vi "Process.vi"(8 "error in":errorcluster, 11 "Measurement.PhotocurrentMapping":refnum<class "Measurement.PhotocurrentMapping.lvclass">) -> (0 "error out":errorcluster, 3 "Measurement.PhotocurrentMapping out":refnum<class "Measurement.PhotocurrentMapping.lvclass">)   [LabVIEW 2017, in "Measurement.PhotocurrentMapping.lvclass"]
doc: "---------------------------------------------------------------\nJKI State Machine Objects™\nhttp://jki.net/state-machine-objects/\nCopyright (C) 2005-2015, JKI <info@jki.net>\nALL RIGHTS RESERVEDJKI State Machine Objects (SMO) 1.0.0.5\nJKI - JKI\nCopyright (c) 2016, JKI"
uses:
  Measurement.PhotocurrentMapping.lvclass
  D:/Program Files (x86)/National Instruments/LabVIEW 2017/vi.lib/JKI/JKI SMO/SMO/SMO.lvclass
  D:/upwork/Laser Measurement Tool/Laser/project/Subsystems/Measurement/Measurement.lvclass
  <vilib>/JKI/JKI SMO/SMO/Typedefs/Parent Call--Enum.ctl
  Measurement/Typedefs/Measurement.State--Enum.ctl
  Typedefs/Measurement.PhotocurrentMapping.State--Enum.ctl
  Typedefs/Results--Cluster.ctl
  Typedefs/Grid--Cluster.ctl
  Typedefs/Position--Cluster.ctl
  Typedefs/Measurement.PhotocurrentMapping.Measured--Data.ctl
  Measurement/Typedefs/PublicEvents--Measurement.Finished.ctl
  Measurement/Typedefs/PublicEvents--Measurement.Initialized.ctl
  Measurement/Typedefs/PublicEvents--Measurement.Escaped.ctl
  <vilib>/Analysis/baseanly.llb/Mean (DBL).vi
  SMU/SMU.lvclass
  D:/upwork/Laser Measurement Tool/Laser/project/Subsystems/MeasuringDevice/MeasuringDevice.lvclass
  LIA/LIA.lvclass
  Measurement/Measurement.lvclass
  <vilib>/JKI/JKI SMO/SMO/SMO.lvclass
  MeasuringDevice/MeasuringDevice.lvclass
  <vilib>/Analysis/NI_AALBase.lvlib
  XYStage/XYStage.lvclass
panel:
  # "Measurement.Photocurrent Mapping\nProcess.vi"
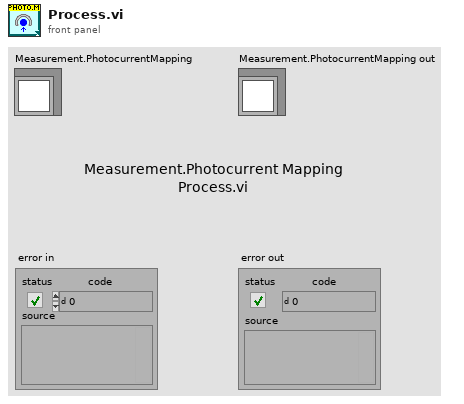
[diagram p1: front panel]
types:
  T1 = typedef "SMO.lvclass/Parent Call--Enum.ctl" = enum16{"Allows parent to run", "Does not request parent to run"}
  T2 = typedef "Measurement.lvclass/Measurement.State--Enum.ctl" = enum16{"Uninitialized", "Initialized", "Started", "Paused", "Stopped"}
  T3 = typedef "Measurement.PhotocurrentMapping.lvclass/Measurement.PhotocurrentMapping.State--Enum.ctl" = enum16{"Stoppped", "Wait for Postition set", "Wait for Measurements"}
  T4 = enum32{"invalid app kind", "Development System", "Run Time System", "Student Edition", "Embedded LabVIEW", "Evaluation", "Custom"}
  T5 = typedef "Measurement.PhotocurrentMapping.lvclass/Position--Cluster.ctl" = cluster{"X":dbl, "Y":dbl}
  T6 = enum32{"Invalid", "Standard", "Closed", "Hidden", "Minimized", "Maximized"}
  T7 = typedef "Measurement.lvclass/PublicEvents--Measurement.Finished.ctl" = bool
  T8 = typedef "Measurement.lvclass/PublicEvents--Measurement.Initialized.ctl" = bool
  T9 = typedef "Measurement.PhotocurrentMapping.lvclass/Dependencies--Cluster.ctl" = cluster{"SMU":refnum<class "SMU.lvclass">, "LIA":refnum<class "LIA.lvclass">, "XYStage":refnum<class "XYStage.lvclass">}
  T10 = typedef "Measurement.PhotocurrentMapping.lvclass/Configuration--Cluster.ctl" = cluster{"Measurement.Type":T11, "Hardware":T12, "Measurement":T19}
  T11 = typedef "Measurement.lvclass/Measurement.Type--Enum.ctl" = enum16{"Free", "I/V Curve", "Wavelength sweeping", "Photocurrent mapping"}
  T12 = typedef "Measurement.PhotocurrentMapping.lvclass/Configuration.Hardware--Cluster.ctl" = cluster{"SMU":T13, "LIA":T15, "XYStage":T17}
  T13 = typedef "Measurement.lvclass/Configuration.SMU--Cluster.ctl" = cluster{"Enable":bool, "SMU Model":string, "Configuration":T14}
  T14 = typedef "SMU.lvclass/Configuration--Cluster.ctl" = cluster{"VISA Resource":string, "Channel":string}
  T15 = typedef "Measurement.lvclass/Configuration.LIA--Cluster.ctl" = cluster{"Enable":bool, "LIA Model":string, "Configuration":T16}
  T16 = typedef "LIA.lvclass/Configuration--Cluster.ctl" = cluster{"VISA Resource":string}
  T17 = typedef "Measurement.lvclass/Configuration.XYStage--Cluster.ctl" = cluster{"Enable":bool, "XYStage Model":string, "Configuration":T18}
  T18 = typedef "XYStage.lvclass/Configuration--Cluster.ctl" = cluster{"Serial Number":string, "X Axis":string, "Y Axis":string, "Real-World Units":string, "Counts per Unit":u32}
  T19 = typedef "Measurement.PhotocurrentMapping.lvclass/Configuration.Measurement--Cluster.ctl" = cluster{"X":T20, "Y":T20, "Accumulation":u16}
  T20 = typedef "Measurement.PhotocurrentMapping.lvclass/Configuration.Axis--Cluster.ctl" = cluster{"Start, units":dbl, "Stop, units":dbl, "Step, units":dbl}
  T21 = typedef "Measurement.PhotocurrentMapping.lvclass/Results--Cluster.ctl" = cluster{"SMU Completed":bool, "LIA Completed":bool, "SMU Measurement":dbl, "LIA Measurement":dbl, "XYStage Completed":bool}
  T22 = typedef "Measurement.PhotocurrentMapping.lvclass/Grid--Cluster.ctl" = cluster{"Positions":T5[][], "X Index":i32, "Y Index":i32, "X Count":u32, "Y Count":u32}
  T23 = cluster{"Core":cluster{"Current VI Reference":refnum<vi>, "Close Panel on Exit?":bool, "error":errorcluster}, "Self Reference":refnum<class "Measurement.PhotocurrentMapping.lvclass">, "Dependencies":T9, "Configuration":T10, "Initialized":bool, "Meas State":T2, "P-Map State":T3, "Next Step":string, "Results":T21, "Grid":T22}
  T24 = cluster{"Current VI Reference":refnum<vi>, "Close Panel on Exit?":bool, "error":errorcluster}
  T25 = typedef "Measurement.PhotocurrentMapping.lvclass/Measurement.PhotocurrentMapping.Measured--Data.ctl" = cluster{"Current, A":dbl, "Magnitude":dbl}
  T26 = typedef "SMO.lvclass/Protected Events.ctl" = cluster{"StopProcesses":refnum<user-event>, "AbortProcesses":refnum<user-event>, "Config Changed":refnum<user-event>, "Dependency":refnum<user-event>}
  T27 = cluster{"Event Registration Refnum":refnum<event-registration>, "Measurement Protected Events":refnum<event-registration>, "SMU Public Events":refnum<event-registration>, "LIA Public Events":refnum<event-registration>, "XYStage Public Events":refnum<event-registration>}
  T28 = typedef "Measurement.lvclass/PublicEvents--Measurement.Escaped.ctl" = bool
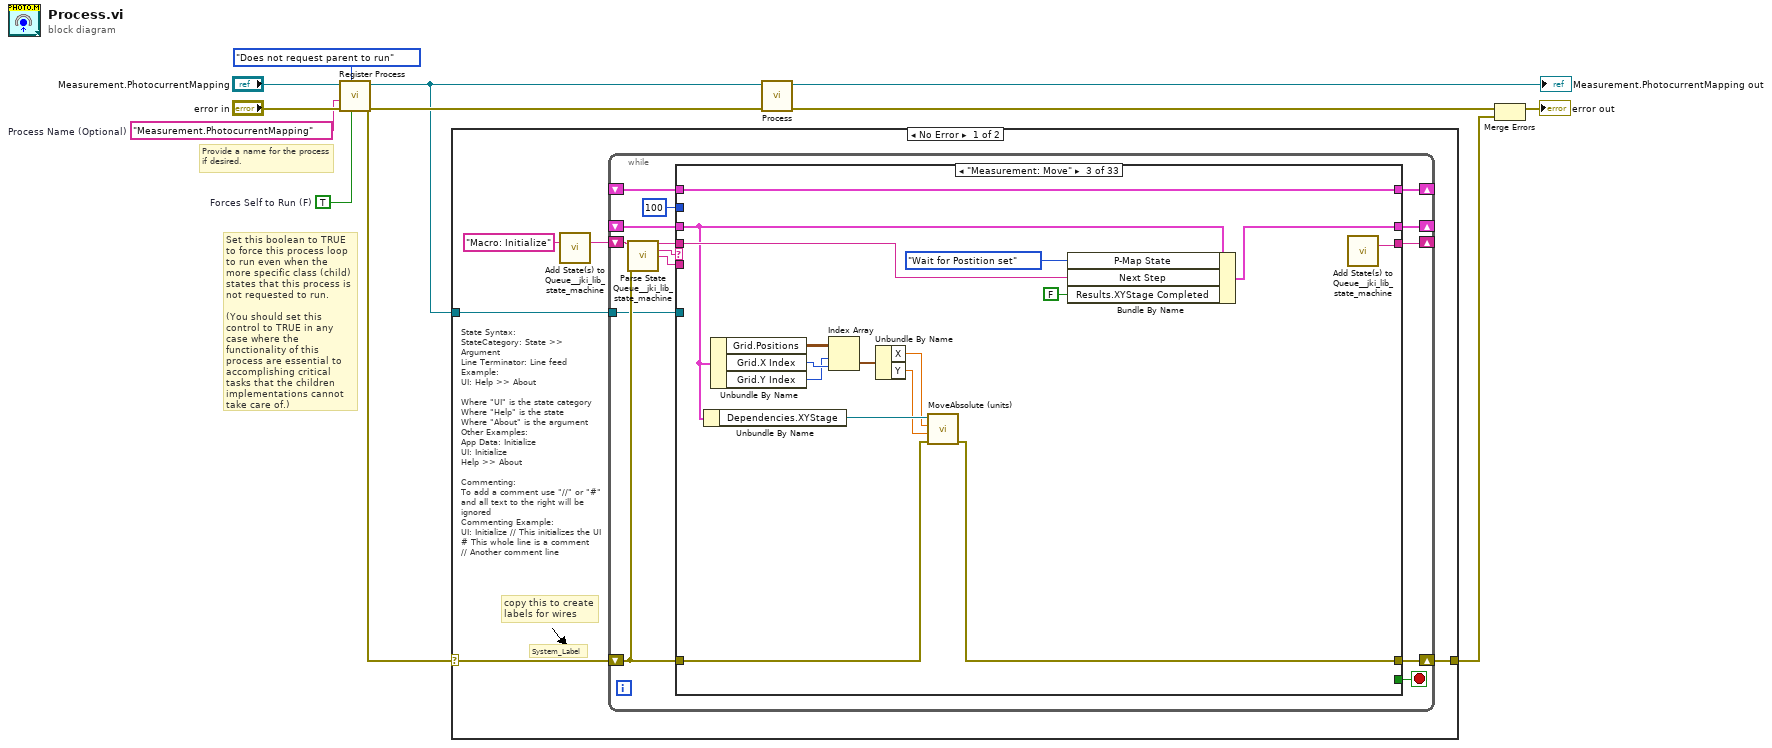
[diagram p0: block diagram]
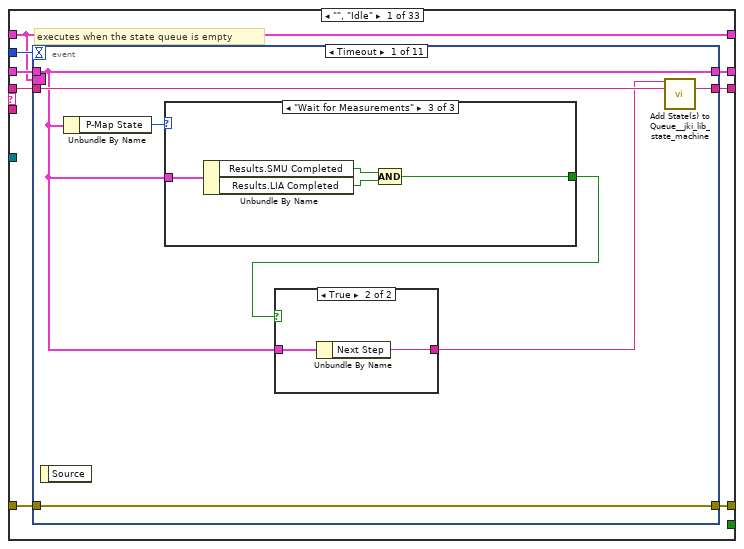
[diagram p2: hidden frame]
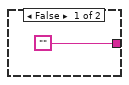
[diagram p3: hidden frame]
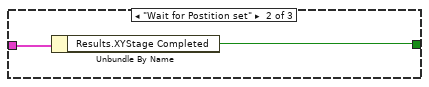
[diagram p5: hidden frame]
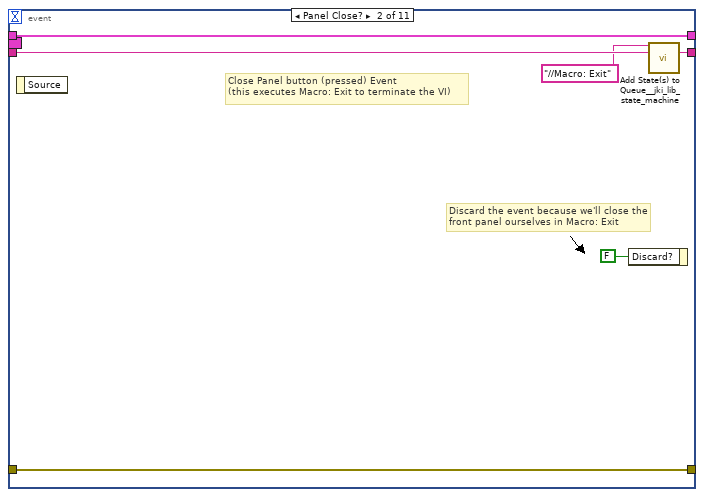
[diagram p6: hidden frame]
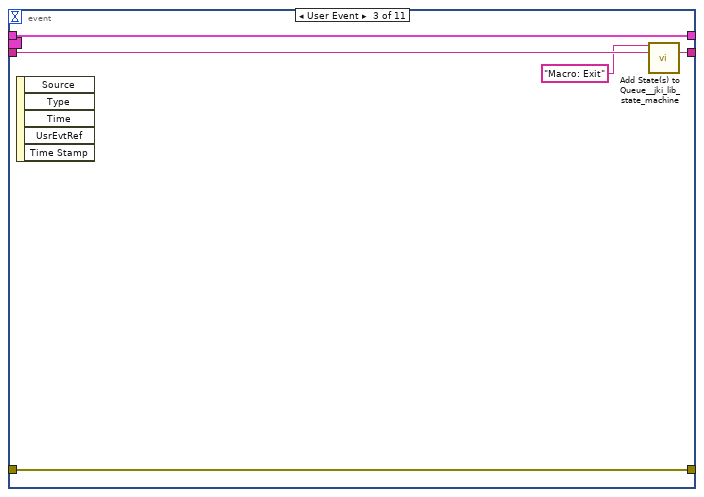
[diagram p7: hidden frame]
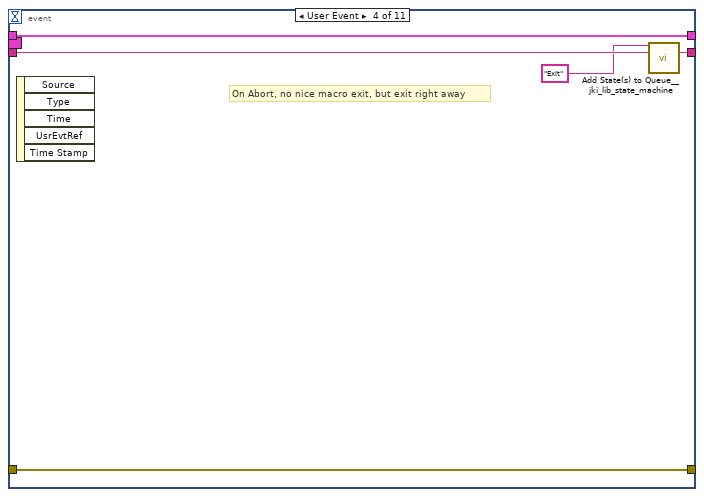
[diagram p8: hidden frame]
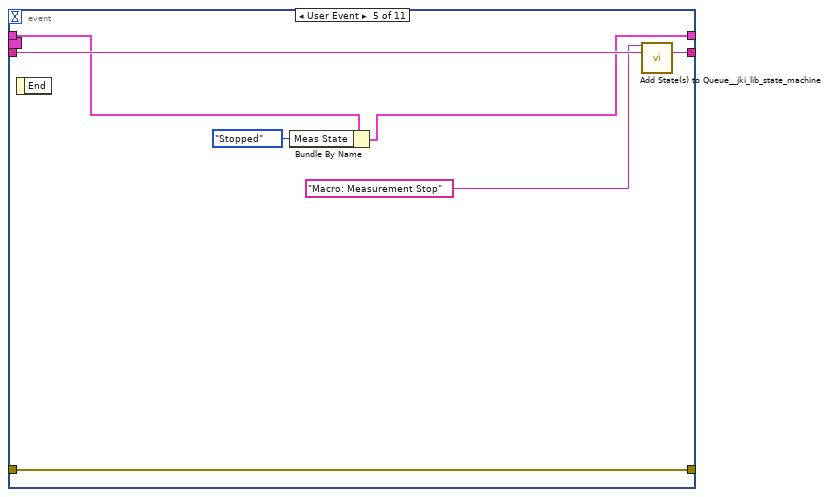
[diagram p9: hidden frame]
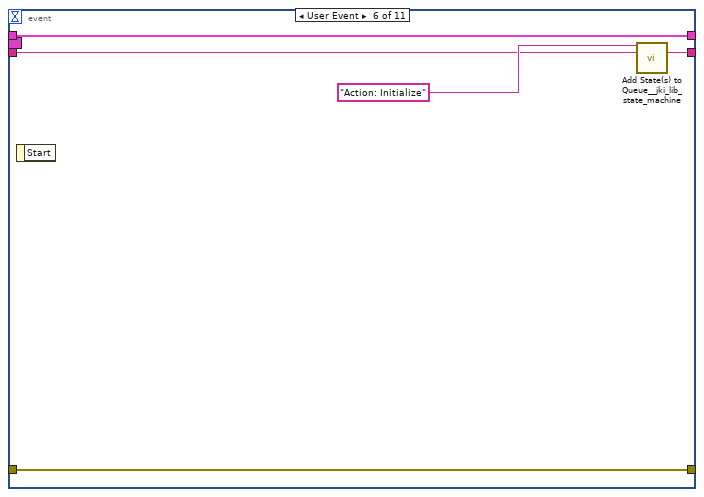
[diagram p10: hidden frame]
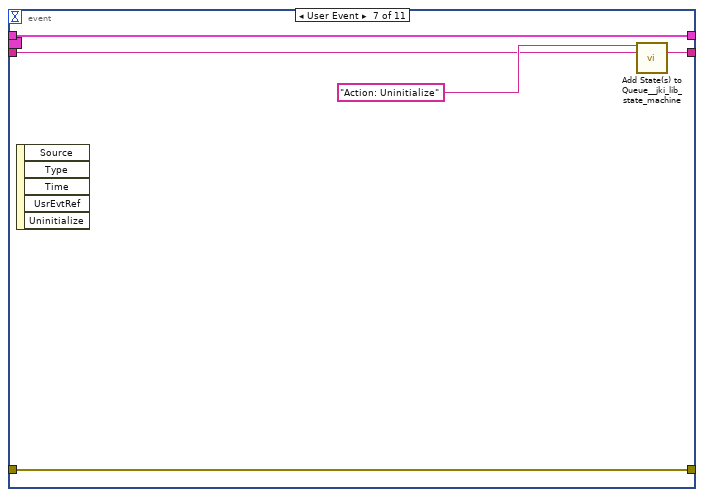
[diagram p11: hidden frame]
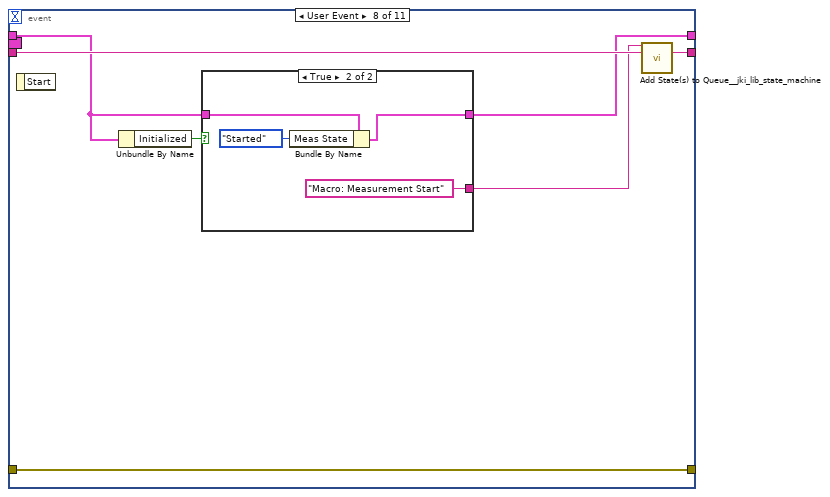
[diagram p12: hidden frame]
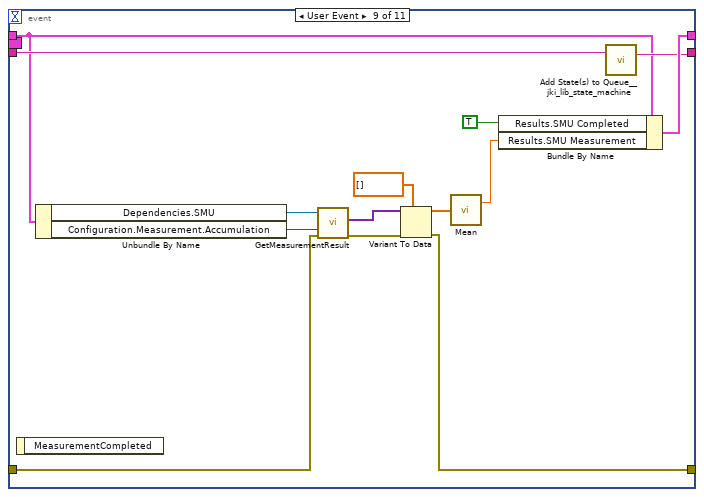
[diagram p14: hidden frame]
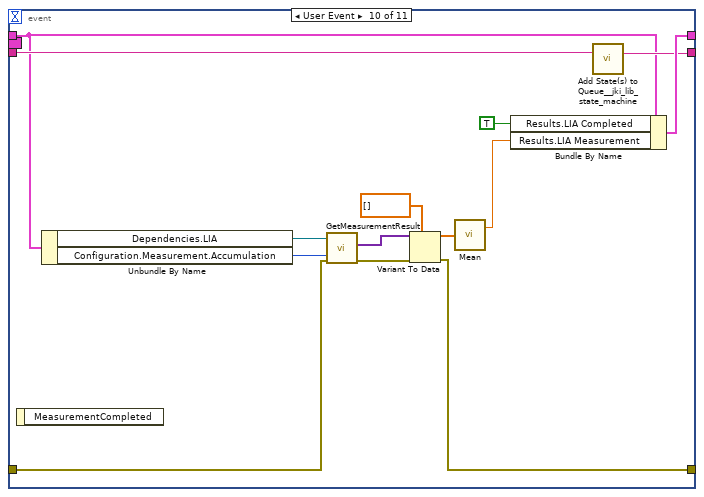
[diagram p15: hidden frame]
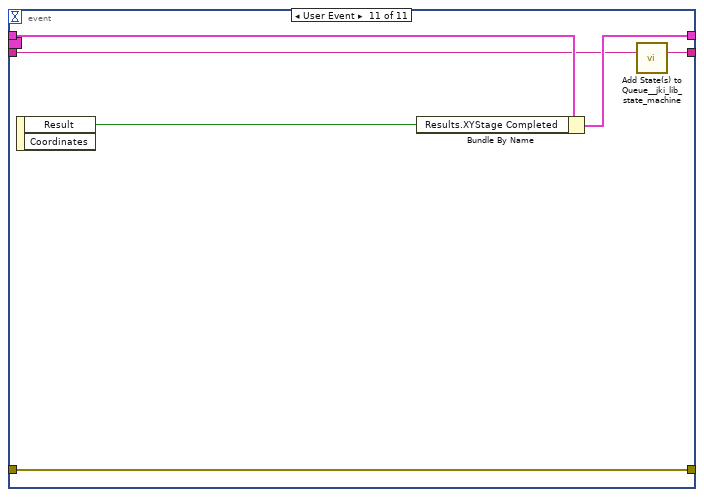
[diagram p16: hidden frame]
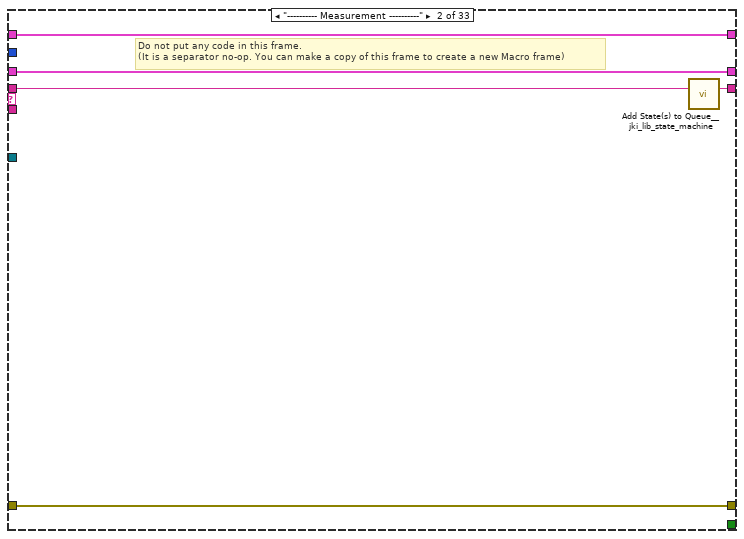
[diagram p17: hidden frame]
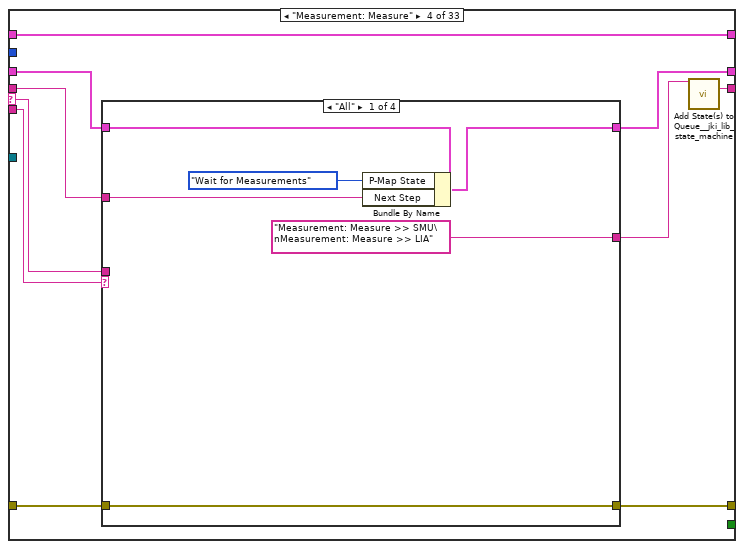
[diagram p18: hidden frame]
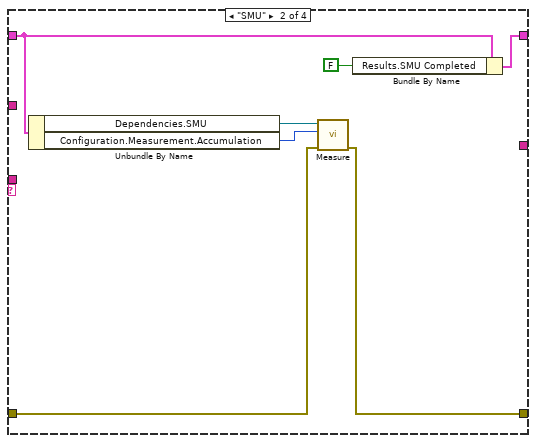
[diagram p19: hidden frame]
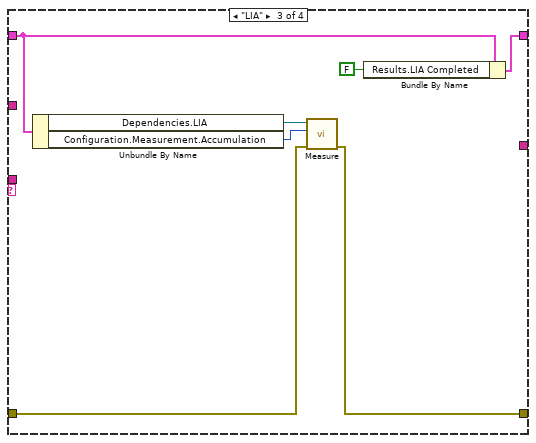
[diagram p20: hidden frame]
diagram:
  w2 = TRUE  # Forces Self to Run (F)
  w1 = "Measurement.PhotocurrentMapping"  # Process Name (Optional)
  # "Provide a name for the process\nif desired."
  # "Set this boolean to TRUE to force this process loop to run even when the more specific class (child) states that this process is not requested to run.\n\n(You should set this control to TRUE in any case where the functionality of this process are essential to accomplishing critical tasks that the children implementations cannot take care of.)"
  n1 = call <vilib>:"Register Process.vi"("Forces Self to Run (F)"=w2, "Parent Call"=Parent_Call--Enum."Does not request parent to run", "error in (no error)"="error in", "Process Name (optional)"=w1, "SMO"="Measurement.PhotocurrentMapping") -> ("error out"=w8:errorcluster, "SMO out"=w7:refnum<class "Measurement.PhotocurrentMapping.lvclass">)  [unwired: 5 in]
  n2 = case shown="No Error" w8 {
    selector: w8 -> [w13 w561]
    tunnel: w7 -> [w14 _]
    tunnel: [w12 w561] -> w4
    frame No Error {
      # "State Syntax:\nStateCategory: State >> Argument\nLine Terminator: Line feed\nExample:\nUI: Help >> About\n\nWhere \"UI\" is the state category\nWhere \"Help\" is the state\nWhere \"About\" is the argument\nOther Examples:\nApp Data: Initialize\nUI: Initialize\nHelp >> About\n\nCommenting:\nTo add a comment use \"//\" or \"#\" and all text to the right will be ignored\nCommenting Example:\nUI: Initialize // This initializes the UI\n# This whole line is a comment\n// Another comment line"
      # "copy this to create labels for wires"
      # "System_Label"
      n3 = call <vilib>:"Add State(s) to Queue__jki_lib_state_machine.vi"("State(s) in (\"\")"="Macro: Initialize") -> ("States Out"=w16:string)  [unwired: 14 in]
      n4 = while {
        shift-right: [w23] -> _
        shift-left: _ -> [w22]
        shift-right: [w26] -> w12
        shift-left: w13 -> [w20]
        shift-right: [w25] -> _
        shift-left: w16 -> [w27]
        tunnel: w14 -> [w19]
        shift-right: [w18] -> _
        shift-left: _ -> [w17]
        stop <- w24 stop-if-true
        n5 = call <vilib>:"Parse State Queue__jki_lib_state_machine.vi"("State Queue"=w27, "Error In (no error)"=w20) -> ("Remaining States"=w29:string, "Current State"=w30:string, "Arguments"=w28:string)  [unwired: 11 in]
        n6 = case shown="\"Measurement: Move\"" w30 {
          selector: w30 -> [_ _ _ w156 _ _ w232 _ _ _ _ _ _ _ _ _ _ _ _ _ _ _ _ _ _ _ _ _ _ _ _ _ _]
          tunnel: w29 -> [w38 w138 w151 w155 w209 w230 w236 w255 w270 w276 w281 w302 w309 w329 w346 w351 w358 w374 w413 w418 w427 w441 w447 w460 w465 w476 w481 w503 w509 w514 w527 w545 w560]
          tunnel: w28 -> [_ _ _ w162 _ _ _ _ _ _ _ _ _ _ _ _ w352 w368 _ _ _ _ _ _ _ _ _ _ _ _ _ _ _]
          tunnel: w22 -> [w36 w135 w150 w158 w198 w227 w234 w246 w261 w272 w278 _ w304 w316 w343 w349 w356 w370 w410 w415 w423 w432 w443 w452 w462 w473 w478 w485 w507 w512 w519 w536 w557]
          tunnel: [w35 w136 w141 w159 w207 w228 w238 w252 w263 w271 w279 w290 w305 w327 w344 w348 w353 w371 w404 w416 w425 w439 w445 w449 w463 w467 w479 w498 w505 w510 w516 w540 w554] -> w26
          tunnel: w20 -> [w34 w136 w142 w160 w207 w228 w237 w252 w258 _ w279 w299 w306 w327 w344 w348 w354 w372 w405 w416 w425 w439 w445 w450 w463 w468 w479 w486 w505 w510 w523 w541 w555]
          tunnel: [w37 w137 w139 w164 w208 w229 w235 w254 w269 w275 w280 w301 w308 w328 w345 w350 w357 w373 w412 w417 w426 w440 w446 w459 w464 w475 w480 w502 w508 w513 w526 w544 w559] -> w25
          tunnel: [_ _ _ _ _ _ _ _ _ TRUE _ _ _ _ _ _ _ _ _ _ _ _ _ _ _ _ _ _ _ _ _ _ _] -> w24
          tunnel: [w33 w135 w153 w157 w195 w227 w234 w253 w260 w272 w278 w300 w304 w315 w343 w349 w356 w370 w410 w415 w423 w432 w443 w453 w462 w473 w478 w485 w507 w512 w518 w539 w557] -> w23
          tunnel: 100 ("Timeout") -> [w32 _ _ _ _ _ _ _ _ _ _ _ _ _ _ _ _ _ _ _ _ _ _ _ _ _ _ _ _ _ _ _ _]
          tunnel: w19 -> [_ _ _ _ _ _ _ _ _ _ _ w297 _ _ _ _ _ _ _ _ _ _ _ _ _ _ _ _ _ _ w524 w542 w556]
          tunnel: [w31 w134 w154 w163 w206 w226 w231 w243 w268 w273 w277 w296 w303 w326 w342 w347 w355 w367 w411 w414 w424 w433 w444 w458 w461 w474 w477 w497 w506 w511 w525 w543 w558] -> w18
          tunnel: w17 -> [w31 w134 w154 w163 w206 w226 w231 w243 w268 w273 w277 w296 w303 w326 w342 w347 w355 w367 w411 w414 w424 w433 w444 w458 w461 w474 w477 _ w506 w511 w525 w543 w558]
          frame "", "Idle" {
            # "executes when the state queue is empty"
            n7 = event shown="[0] Timeout" {
              selector: w31 -> [_ _ _ _ _ _ _ _ _ _ _]
              dyn-events: _ -> [_ _ _ _ _ _ _ _ _ _ _]
              timeout: w32 -> [_ _ _ _ _ _ _ _ _ _ _]
              tunnel: w38 -> [w45 w60 w65 w70 w76 w78 w83 w93 w111 w125 w130]
              tunnel: [w44 w59 w64 w69 w77 w80 w85 w94 w112 w126 w131] -> w37
              tunnel: w36 -> [w40 w57 w62 w67 w73 w81 w86 w89 w110 w121 w133]
              tunnel: [w43 w58 w63 w68 w75 w82 w87 w92 w105 w119 w128] -> w35
              tunnel: w34 -> [w43 w58 w63 w68 w75 w82 w87 w92 w108 w120 w128]
              tunnel: [w40 w57 w62 w67 w72 w81 w86 w88 w113 w127 w132] -> w33
              event Timeout {
                n8 = event-data() -> ()  [unwired: 1 in, 1 out]
                n9 = Unbundle By Name(w40) -> ("P-Map State"=w42:T3)
                n10 = case shown="\"Wait for Measurements\"" w42 {
                  tunnel: w40 -> [_ w50 w54]
                  tunnel: [_ w49 w52] -> w41
                  frame "Stoppped", Default {
                  }
                  frame "Wait for Postition set" {
                    n11 = Unbundle By Name(w50) -> ("Results.XYStage Completed"=w49:bool)
                  }
                  frame "Wait for Measurements" {
                    n12 = Unbundle By Name(w54) -> ("Results.SMU Completed"=w53:bool, "Results.LIA Completed"=w51:bool)
                    n13 = Compound Arithmetic op=AND(w53, w51) -> (w52:bool)
                  }
                }
                n14 = case shown="True" w41 {
                  tunnel: w40 -> [_ w48]
                  tunnel: ["" w47] -> w39
                  frame False {
                  }
                  frame True {
                    n15 = Unbundle By Name(w48) -> ("Next Step"=w47:string)
                  }
                }
                n16 = call <vilib>:"Add State(s) to Queue__jki_lib_state_machine.vi"("State(s) in Front (\"\")"=w39, "State(s) in (\"\")"=w45) -> ("States Out"=w44:string)  [unwired: 13 in]
              }
              event Panel Close? {
                # "Discard the event because we'll close the front panel ourselves in Macro: Exit"
                # "Close Panel button (pressed) Event\n(this executes Macro: Exit to terminate the VI)"
                n17 = event-data() -> ()  [unwired: 1 in, 1 out]
                n18 = event-data("Discard?"=FALSE) -> ()  [unwired: 1 in, 1 out]
                n19 = call <vilib>:"Add State(s) to Queue__jki_lib_state_machine.vi"("State(s) in Front (\"\")"="//Macro: Exit", "State(s) in (\"\")"=w60) -> ("States Out"=w59:string)  [unwired: 13 in]
              }
              event User Event {
                n20 = event-data() -> ()  [unwired: 1 in, 5 out]
                n21 = call <vilib>:"Add State(s) to Queue__jki_lib_state_machine.vi"("State(s) in Front (\"\")"="Macro: Exit", "State(s) in (\"\")"=w65) -> ("States Out"=w64:string)  [unwired: 13 in]
              }
              event User Event {
                # "On Abort, no nice macro exit, but exit right away"
                n22 = event-data() -> ()  [unwired: 1 in, 5 out]
                n23 = call <vilib>:"Add State(s) to Queue__jki_lib_state_machine.vi"("State(s) in Front (\"\")"="Exit", "State(s) in (\"\")"=w70) -> ("States Out"=w69:string)  [unwired: 13 in]
              }
              event User Event {
                n24 = event-data() -> ()  [unwired: 1 in, 1 out]
                n25 = Bundle By Name(cluster=w73, "Meas State"=Measurement.State--Enum."Stopped") -> (w72:T23)
                n26 = call <vilib>:"Add State(s) to Queue__jki_lib_state_machine.vi"("State(s) in Front (\"\")"="Macro: Measurement Stop", "State(s) in (\"\")"=w76) -> ("States Out"=w77:string)  [unwired: 13 in]
              }
              event User Event {
                n27 = event-data() -> ()  [unwired: 1 in, 1 out]
                n28 = call <vilib>:"Add State(s) to Queue__jki_lib_state_machine.vi"("State(s) in Front (\"\")"="Action: Initialize", "State(s) in (\"\")"=w78) -> ("States Out"=w80:string)  [unwired: 13 in]
              }
              event User Event {
                n29 = event-data() -> ()  [unwired: 1 in, 5 out]
                n30 = call <vilib>:"Add State(s) to Queue__jki_lib_state_machine.vi"("State(s) in Front (\"\")"="Action: Uninitialize", "State(s) in (\"\")"=w83) -> ("States Out"=w85:string)  [unwired: 13 in]
              }
              event User Event {
                n31 = event-data() -> ()  [unwired: 1 in, 1 out]
                n32 = Unbundle By Name(w89) -> ("Initialized"=w90:bool)
                n33 = case shown="True" w90 {
                  tunnel: [_ "Macro: Measurement Start"] -> w91
                  tunnel: w89 -> [w95 w98]
                  tunnel: [w95 w96] -> w88
                  frame False {
                  }
                  frame True {
                    n34 = Bundle By Name(cluster=w98, "Meas State"=Measurement.State--Enum."Started") -> (w96:T23)
                  }
                }
                n35 = call <vilib>:"Add State(s) to Queue__jki_lib_state_machine.vi"("State(s) in Front (\"\")"=w91, "State(s) in (\"\")"=w93) -> ("States Out"=w94:string)  [unwired: 13 in]
              }
              event User Event {
                n36 = event-data() -> ()  [unwired: 1 in, 1 out]
                n37 = Unbundle By Name(w110) -> ("Dependencies.SMU"=w109:refnum<class "SMU.lvclass">, "Configuration.Measurement.Accumulation"=w101:u16)
                n38 = call "GetMeasurementResult.vi"("error in (no error)"=w108, "Count (1)"=w101, "MeasuringDevice in"=w109) -> ("error out"=w106:errorcluster, "Result"=w107:variant[])  [unwired: 6 in, 1 out]
                n39 = Variant To Data(error in=w106, type=dbl[] [], Variant=w107) -> (data=w103:dbl[], error out=w105:errorcluster)
                n40 = call-poly <vilib>:"Mean.vi"("X"=w103) -> ("mean"=w102:dbl)  [unwired: 1 out]
                n41 = Bundle By Name(cluster=w110, "Results.SMU Completed"=TRUE ("OPA Wavelength"), "Results.SMU Measurement"=w102) -> (w113:T23)
                n42 = call <vilib>:"Add State(s) to Queue__jki_lib_state_machine.vi"("State(s) in (\"\")"=w111) -> ("States Out"=w112:string)  [unwired: 14 in]
              }
              event User Event {
                n43 = event-data() -> ()  [unwired: 1 in, 1 out]
                n44 = Unbundle By Name(w121) -> ("Dependencies.LIA"=w124:refnum<class "LIA.lvclass">, "Configuration.Measurement.Accumulation"=w115:u16)
                n45 = call "GetMeasurementResult.vi"("error in (no error)"=w120, "Count (1)"=w115, "MeasuringDevice in"=w124) -> ("error out"=w122:errorcluster, "Result"=w123:variant[])  [unwired: 6 in, 1 out]
                n46 = Variant To Data(error in=w122, type=dbl[] [], Variant=w123) -> (data=w118:dbl[], error out=w119:errorcluster)
                n47 = call-poly <vilib>:"Mean.vi"("X"=w118) -> ("mean"=w116:dbl)  [unwired: 1 out]
                n48 = Bundle By Name(cluster=w121, "Results.LIA Completed"=TRUE ("OPA Wavelength"), "Results.LIA Measurement"=w116) -> (w127:T23)
                n49 = call <vilib>:"Add State(s) to Queue__jki_lib_state_machine.vi"("State(s) in (\"\")"=w125) -> ("States Out"=w126:string)  [unwired: 14 in]
              }
              event User Event {
                n50 = event-data() -> ("Result"=w129:bool)  [unwired: 1 in, 1 out]
                n51 = Bundle By Name(cluster=w133, "Results.XYStage Completed"=w129) -> (w132:T23)
                n52 = call <vilib>:"Add State(s) to Queue__jki_lib_state_machine.vi"("State(s) in (\"\")"=w130) -> ("States Out"=w131:string)  [unwired: 14 in]
              }
            }
          }
          frame "---------- Measurement ----------" {
            # "Do not put any code in this frame.\n(It is a separator no-op. You can make a copy of this frame to create a new Macro frame)"
            n53 = call <vilib>:"Add State(s) to Queue__jki_lib_state_machine.vi"("State(s) in (\"\")"=w138) -> ("States Out"=w137:string)  [unwired: 14 in]
          }
          frame "Measurement: Move" {
            n54 = Unbundle By Name(w150) -> ("Dependencies.XYStage"=w149:refnum<class "XYStage.lvclass">)
            n55 = Unbundle By Name(w150) -> ("Grid.Positions"=w148:T5[][], "Grid.X Index"=w147:i32, "Grid.Y Index"=w146:i32)
            n56 = Index Array(array=w148, index (row)=w146, index (col)=w147) -> (element=w145:T5)
            n57 = Unbundle By Name(w145) -> ("X"=w144:dbl, "Y"=w143:dbl)
            n58 = call "MoveAbsolute (units).vi"("error in (no error)"=w142, "Y, units"=w143, "X, units"=w144, "XYStage"=w149) -> ("error out"=w141:errorcluster)  [unwired: 6 in, 1 out]
            n59 = Bundle By Name(cluster=w150, "P-Map State"=Measurement.PhotocurrentMapping.State--Enum."Wait for Postition set" ("W-Sweep State"), "Next Step"=w151, "Results.XYStage Completed"=FALSE) -> (w153:T23)
            n60 = call <vilib>:"Add State(s) to Queue__jki_lib_state_machine.vi"() -> ("States Out"=w139:string)  [unwired: 15 in]
          }
          frame "Measurement: Measure" {
            n61 = case shown="\"All\"" w162 {
              selector: w162 -> [_ _ _ w188]
              tunnel: ["Measurement: Measure >> SMU\nMeasurement: Measure >> LIA" ("Next Step") _ _ _] -> w161
              tunnel: w160 -> [w169 w176 w183 w187]
              tunnel: [w169 w175 w182 w186] -> w159
              tunnel: w158 -> [w168 w171 w178 w185]
              tunnel: [w167 w174 w181 w185] -> w157
              tunnel: w156 -> [_ _ _ w189]
              tunnel: w155 -> [w165 _ _ _]
              frame "All" {
                n62 = Bundle By Name(cluster=w168, "P-Map State"=Measurement.PhotocurrentMapping.State--Enum."Wait for Measurements" ("W-Sweep State"), "Next Step"=w165) -> (w167:T23)
              }
              frame "SMU" {
                n63 = Unbundle By Name(w171) -> ("Dependencies.SMU"=w177:refnum<class "SMU.lvclass">, "Configuration.Measurement.Accumulation"=w173:u16)
                n64 = call "Measure.vi"("error in (no error)"=w176, "Count (1)"=w173, "MeasuringDevice"=w177) -> ("error out"=w175:errorcluster)  [unwired: 6 in, 2 out]
                n65 = Bundle By Name(cluster=w171, "Results.SMU Completed"=FALSE ("SMU Completed")) -> (w174:T23)
              }
              frame "LIA" {
                n66 = Unbundle By Name(w178) -> ("Dependencies.LIA"=w184:refnum<class "LIA.lvclass">, "Configuration.Measurement.Accumulation"=w180:u16)
                n67 = call "Measure.vi"("error in (no error)"=w183, "Count (1)"=w180, "MeasuringDevice"=w184) -> ("error out"=w182:errorcluster)  [unwired: 6 in, 2 out]
                n68 = Bundle By Name(cluster=w178, "Results.LIA Completed"=FALSE ("SMU Completed")) -> (w181:T23)
              }
              frame "Error", Default {
                w191 = "\r\n"
                n69 = Concatenate Strings("Nonexistent state caused" ("source"), w191, w189, w191, w188) -> (w190:string)
                n70 = call <vilib>:"Error Cluster From Error Code.vi"("error in (no error)"=w187, "error message (\"\")"=w190, "error code (0)"=-8000 ("code")) -> ("error out"=w186:errorcluster)  [unwired: 6 in]
              }
            }
            n71 = call <vilib>:"Add State(s) to Queue__jki_lib_state_machine.vi"("State(s) in Front (\"\")"=w161) -> ("States Out"=w164:string)  [unwired: 14 in]
          }
          frame "Measurement: Next Step" {
            n72 = Unbundle By Name(w198) -> ("Grid.X Index"=w204:i32, "Grid.X Count"=w203:u32, "Grid.Y Index"=w201:i32, "Grid.Y Count"=w200:u32)
            n73 = Increment(x=w204) -> (x+1=w199:i32)
            n74 = Greater Or Equal?(x=w199, y=w203) -> (x >= y?=w202:bool)
            n75 = case shown="True" w202 {
              tunnel: w201 -> [w211 w219]
              tunnel: w200 -> [_ w218]
              tunnel: w199 -> [w212 _]
              tunnel: [w212 0] -> w197
              tunnel: [w211 w214] -> w196
              tunnel: [TRUE w213] -> w194
              frame False {
              }
              frame True {
                n76 = Increment(x=w219) -> (x+1=w215:i32)
                n77 = Greater Or Equal?(x=w215, y=w218) -> (x >= y?=w216:bool)
                n78 = case shown="True" w216 {
                  tunnel: w215 -> [w221 _]
                  tunnel: [w221 0] -> w214
                  tunnel: [TRUE FALSE] -> w213
                  frame False {
                  }
                  frame True {
                  }
                }
              }
            }
            n79 = case shown="True" w194 {
              tunnel: ["Macro: Measurement Stop" "Macro: Measurement Start"] -> w205
              frame False {
                # "Stop measurement"
              }
              frame True {
                # "Go to next wavelength"
              }
            }
            n80 = Bundle By Name(cluster=w198, "Grid.X Index"=w197, "Grid.Y Index"=w196) -> (w195:T23)
            n81 = call <vilib>:"Add State(s) to Queue__jki_lib_state_machine.vi"("State(s) in Front (\"\")"=w205, "State(s) in (\"\")"=w209) -> ("States Out"=w208:string)  [unwired: 13 in]
          }
          frame "---------- Core ----------" {
            # "Do not put any code in this frame.\n(it is a separator no-op)"
            n82 = call <vilib>:"Add State(s) to Queue__jki_lib_state_machine.vi"("State(s) in (\"\")"=w230) -> ("States Out"=w229:string)  [unwired: 14 in]
          }
          frame Default {
            w241 = 42 items=["No error", "Argument error", "Memory is full", "Out of zone", "End of file", "File already open", "Generic file I/O error", "File not found", "File permission error", "Disk is full", "Duplicate path", "Too many files open", "System feature not enabled", "Resource file not found", "Cannot add resource", "Resource not found", "Image not found", "Image memory error", "Pen does not exist", "Config type invalid", "Config token not found", "Config parse error", "Config memory error", "Bad external code format", "Bad external code offset", "External code not present", "Null window", "Destroy window error", "Null menu", "Print aborted", "Bad print record", "Print driver error", "Windows error during printing", "Memory error during printing", "Print dialog error", "Generic print error", "Invalid device refnum", "Device not found", "Device parameter error", "Device unit error", "Cannot open device", "Device call aborted", "Generic error", "Cancelled by user", "Object ID too low", "Object ID too high", "Object not in heap", "Unknown heap", "Unknown object (invalid DefProc)", "Unknown object (DefProc not in table)", "Message out of range", "Invalid (null) method", "Unknown message", "Manager call not supported", "Bad address", "Network operation in progress", "Network operation timed out", "Connection is busy", "Network attribute not supported", "Network error", "Address in use", "System out of memory", "Connection aborted", "Connection refused", "Not connected", "Already connected", "Connection closed", "Initialization error (interapplication manager)", "Bad occurrence", "Wait on unbound occurrence handler", "Occurrence queue overflow", "Datalog type conflict", "Unused", "Unrecognized type (interapplication manager)", "Memory corrupt", "Failed to make temporary DLL", "Old CIN version", "Drag socket not found", "Failed to load drop-object", "Failed to register OLE object", "Failed to release OLE object", "Format specifier type mismatch", "Unknown format specifier", "Too few format specifiers", "Too many format specifiers", "Scan failed", "Newer CIN version", "Error converting to variant", "Runtime menu error", "Password tampered", "Variant attribute not found", "Incompatible variant data type", "Event data is not available", "Event Store is not present", "Occurrence is not found", "Event Queue is not created", "Event info is not available", "Refnum passed is NULL", "Error retrieving Class GUID", "Error retrieving CoClass GUID", "Error retrieving TypeLib GUID.", "Bad built application magic bytes.", "Specific driver is different from the specific driver associated with the Logical Name.", "There is no session opened to the class driver.", "Max Error", "MAX - Error with config objects", "MAX - Error loading configuration", "MAX - Group not supported"]
            # "Current State"
            # "Do not delete, rename, or modify this frame.\n(this is used to capture unhandled states and typos)"
            # "Handle mistyped state name (developer tool)"
            n83 = Format Into String(format string="Software Exception: Unhandled State \"%s\"." ("message"), error in=w237, w232) -> (resulting string=w240:string, error out=w239:errorcluster)  [unwired: 1 in]
            n84 = call <vilib>:"Error Cluster From Error Code.vi"("show call chain? (False)"=TRUE, "error in (no error)"=w239, "error message (\"\")"=w240, "error code (0)"=w241) -> ("error out"=w238:errorcluster)  [unwired: 5 in]
            n85 = call <vilib>:"Add State(s) to Queue__jki_lib_state_machine.vi"("State(s) in (\"\")"=w236) -> ("States Out"=w235:string)  [unwired: 14 in]
          }
          frame "Initialize Core Data" {
            # "Do not delete, rename, or modify this frame.\n(this is used to determine panel behavior on exit)"
            # "originally closed?"
            # "exe?"
            # "If panel starts closed or is an EXE, then close it when we exit"
            n86 = property class="VI"() -> ("Front Panel.Open"=w251:bool)  [unwired: 2 in, 2 out]
            n87 = property class="App"() -> ("App.Kind"=w250:T4)  [unwired: 2 in, 2 out]
            n88 = control-ref of="Current VI Reference"() -> (w244:refnum<vi>)
            n89 = Not(x=w251) -> (.not. x?=w248:bool)
            n90 = Equal?(x=w250, y=T4."Run Time System" ("Application:Kind")) -> (x = y?=w247:bool)
            n91 = Or(x=w248, y=w247) -> (x .or. y?=w245:bool)
            n92 = Bundle By Name(cluster=w246, "Core.Current VI Reference"=w244, "Core.Close Panel on Exit?"=w245) -> (w253:T23)
            n93 = call <vilib>:"Add State(s) to Queue__jki_lib_state_machine.vi"("State(s) in (\"\")"=w255) -> ("States Out"=w254:string)  [unwired: 14 in]
          }
          frame "Error Handler" {
            w263 = errorcluster {"status"=FALSE, "code"=0, "source"=""}  # No error
            (unwired) "Exit"
            # "Overwrite this method to handle errors and pass to parent if not handled. Parent will fire a public event if the error is not handled up the chain of classes."
            # "Handle any errors here.\nYou can also output any states to clean-up after errors occur"
            n94 = Unbundle By Name(w261) -> ("Self Reference"=w267:refnum<class "Measurement.PhotocurrentMapping.lvclass">)
            n95 = call <vilib>:"Simple Error Handler.vi"("error in (no error)"=w258) -> ("error out"=w257:errorcluster)  [unwired: 4 in, 4 out]
            n96 = call-dynamic "Handle Error.vi"("Stop on Unhandled Error (T)"=TRUE, "error in"=w257, "Measurement"=w267) -> ("handling error"=w264:errorcluster, "Unhandled error"=w262:errorcluster)  [unwired: 6 in, 1 out]
            n97 = Bundle By Name(cluster=w261, "Core.error"=w262) -> (w260:T23)
            n98 = Select(t="Action: Uninitialize\nAction: Escape", s=w264, f="") -> (s? t:f=w265:string)
            n99 = call <vilib>:"Add State(s) to Queue__jki_lib_state_machine.vi"("State(s) in Front (\"\")"=w265, "State(s) in (\"\")"=w270) -> ("States Out"=w269:string)  [unwired: 13 in]
          }
          frame "Exit" {
            # "Do not put any code in this frame.\n(No errors that occur here will be handled.)"
            n100 = Unbundle By Name(w272) -> ("Core.error"=w271:errorcluster)
            n101 = call <vilib>:"Add State(s) to Queue__jki_lib_state_machine.vi"("State(s) in (\"\")"=w276) -> ("States Out"=w275:string)  [unwired: 14 in]
          }
          frame "---------- Data ----------" {
            # "Do not put any code in this frame.\n(It is a separator no-op. You can make a copy of this frame to create a new Data frame)"
            n102 = call <vilib>:"Add State(s) to Queue__jki_lib_state_machine.vi"("State(s) in (\"\")"=w281) -> ("States Out"=w280:string)  [unwired: 14 in]
          }
          frame "Data: Initialize" {
            w282 = T22 {"Positions"=[], "X Index"=0, "Y Index"=0, "X Count"=0, "Y Count"=0}  # Grid
            w283 = T21 {"SMU Completed"=FALSE, "LIA Completed"=FALSE, "SMU Measurement"=0.0, "LIA Measurement"=0.0, "XYStage Completed"=FALSE}  # Results
            w284 = ""  # Next Step
            w285 = Measurement.PhotocurrentMapping.State--Enum."Stoppped"  # P-Map State
            w286 = FALSE  # Initialized
            w287 = Measurement.State--Enum."Uninitialized"  # Meas State
            w295 = T24 {"Current VI Reference"=refnum, "Close Panel on Exit?"=FALSE, "error"={"status"=FALSE, "code"=0, "source"=""}}  # Core
            w298 = refnum<class "Measurement.PhotocurrentMapping.lvclass"> refnum  # Self Reference
            # "Configuration"
            # "Dependencies"
            # "do not delete - used by framework"
            # "Data names and types of shift register data are defined by this bundle."
            # "Initialize the shift-register data, here.\n(data names are defined by what you wire into the bundle function)"
            n103 = Variant To Data(error in=w299, type=w298, Variant=w297) -> (data=w294:refnum<class "Measurement.PhotocurrentMapping.lvclass">, error out=w293:errorcluster)
            n104 = call "Measurement.PhotocurrentMapping.GetStaticDependencies.vi"("error in (no error)"=w293, "Measurement.PhotocurrentMapping in"=w294) -> ("error out"=w291:errorcluster, "Dependencies"=w289:T9, "Measurement.PhotocurrentMapping out"=w292:refnum<class "Measurement.PhotocurrentMapping.lvclass">)  [unwired: 7 in]
            n105 = call "Measurement.PhotocurrentMapping.GetConfiguration.vi"("error in (no error)"=w291, "Measurement.PhotocurrentMapping"=w292) -> ("error out"=w290:errorcluster, "Configuration"=w288:T10)  [unwired: 7 in, 1 out]
            n106 = Bundle("Core"=w295, "Self Reference"=w294, "Dependencies"=w289, "Configuration"=w288, "Initialized"=w286, "Meas State"=w287, "P-Map State"=w285, "Next Step"=w284, "Results"=w283, "Grid"=w282) -> (w300:T23)  [unwired: 1 in]
            n107 = call <vilib>:"Add State(s) to Queue__jki_lib_state_machine.vi"("State(s) in (\"\")"=w302) -> ("States Out"=w301:string)  [unwired: 14 in]
          }
          frame "Data: Cleanup" {
            # "Cleanup any data and references, here.\n(this is called automatically, by the Macro: Exit)"
            n108 = Unbundle By Name(w304) -> ("Core.Current VI Reference"=w307:refnum<vi>)
            n109 = Close Reference(reference=w307, error in (no error)=w306) -> (error out=w305:errorcluster)
            n110 = call <vilib>:"Add State(s) to Queue__jki_lib_state_machine.vi"("State(s) in (\"\")"=w309) -> ("States Out"=w308:string)  [unwired: 14 in]
          }
          frame "Data: Initialize Grid" {
            n111 = Unbundle By Name(w316) -> ("Configuration.Measurement.X.Start, units"=w325:dbl, "Configuration.Measurement.X.Stop, units"=w324:dbl, "Configuration.Measurement.X.Step, units"=w323:dbl, "Configuration.Measurement.Y.Start, units"=w322:dbl, "Configuration.Measurement.Y.Stop, units"=w321:dbl, "Configuration.Measurement.Y.Step, units"=w320:dbl)
            n112 = call "Create Linear Vector.vi"("Step"=w323, "Stop"=w324, "Start"=w325) -> ("Count"=w314:i32, "Vector"=w319:dbl[])  [unwired: 6 in, 1 out]
            n113 = call "Create Linear Vector.vi"("Step"=w320, "Stop"=w321, "Start"=w322) -> ("Count"=w313:i32, "Vector"=w318:dbl[])  [unwired: 6 in, 1 out]
            n114 = for {
              tunnel: w319 -> [w334]
              tunnel: w318 -> [w335] mode=indexing
              shift-right: [w331] -> w310
              shift-left: T5[][] [] ("Grid.Positions") -> [w332]
              n115 = for {
                tunnel: w335 -> [w340]
                tunnel: w334 -> [w339] mode=indexing
                shift-right: [w337] -> w330
                shift-left: T5[] [{"X"=0.0, "Y"=0.0}] -> [w338]
                w341 = T5 {"X"=0.0, "Y"=0.0}  # Position
                n116 = Bundle By Name(cluster=w341, "X"=w339, "Y"=w340) -> (w336:T5)
                n117 = Build Array (concatenate)(w338, w336) -> (w337:T5[])
              }
              n118 = Build Array (concatenate)(w332, w330) -> (w331:T5[][])
            }
            n119 = Bundle By Name(cluster=w316, "Grid.Positions"=w310, "Grid.X Index"=u32 0, "Grid.Y Index"=u32 0, "Grid.X Count"=w314, "Grid.Y Count"=w313) -> (w315:T23)
            n120 = call <vilib>:"Add State(s) to Queue__jki_lib_state_machine.vi"("State(s) in (\"\")"=w329) -> ("States Out"=w328:string)  [unwired: 14 in]
          }
          frame "---------- UI ----------" {
            # "Do not put any code in this frame.\n(It is a separator no-op. You can make a copy of this frame to create a new UI frame)"
            n121 = call <vilib>:"Add State(s) to Queue__jki_lib_state_machine.vi"("State(s) in (\"\")"=w346) -> ("States Out"=w345:string)  [unwired: 14 in]
          }
          frame "UI: Initialize" {
            # "Initialize the User Interface, here.\n(this is called automatically, by the Macro: Init)"
            n122 = call <vilib>:"Add State(s) to Queue__jki_lib_state_machine.vi"("State(s) in (\"\")"=w351) -> ("States Out"=w350:string)  [unwired: 14 in]
          }
          frame "UI: Cursor Set" {
            # "Argument"
            # "Initialize the User Interface, here.\n(this is called automatically, by the Macro: Init)"
            n123 = disable-structure shown="Default" {
              disable-tunnel: w354 -> [w359 w362]
              disable-tunnel: [w359 w361] -> w353
              disable-tunnel: w352 -> [_ w360]
              frame condition #0 {
              }
              frame condition #1 (active) {
                n124 = case shown="\"Busy\"" w360 {
                  tunnel: w362 -> [w364 w366]
                  tunnel: [w363 w365] -> w361
                  frame "Idle", Default {
                    n125 = call <vilib>:"Unset Busy.vi"("error in (no error)"=w364) -> ("error out"=w363:errorcluster)  [unwired: 10 in]
                  }
                  frame "Busy" {
                    n126 = call <vilib>:"Set Busy.vi"("error in (no error)"=w366) -> ("error out"=w365:errorcluster)  [unwired: 9 in, 1 out]
                  }
                }
              }
            }
            n127 = call <vilib>:"Add State(s) to Queue__jki_lib_state_machine.vi"("State(s) in (\"\")"=w358) -> ("States Out"=w357:string)  [unwired: 14 in]
          }
          frame "UI: Front Panel State" {
            # "Argument"
            # "Set Front Panel Open or Closed\n(Usage: \"UI: Front Panel State >> Open|Close\")"
            n128 = Unbundle By Name(w370) -> ("Core.Current VI Reference"=w369:refnum<vi>)
            n129 = disable-structure shown="Default" {
              disable-tunnel: w372 -> [w378 w401]
              disable-tunnel: [w377 w401] -> w371
              disable-tunnel: w369 -> [w376 _]
              disable-tunnel: w368 -> [w375 _]
              frame condition #0 (active) {
                n130 = case shown="\"Open\", Default" w375 {
                  tunnel: w378 -> [w382 w395]
                  tunnel: [w384 w396] -> w377
                  tunnel: w376 -> [w383 w393]
                  frame "Open", Default {
                    n131 = property class="VI"(reference=w383, error in=w382) -> (reference out=w380:refnum<vi>, error out=w381:errorcluster, "FP.State"=w379:T6)
                    n132 = case shown="\"Closed\"" w379 {
                      tunnel: [w387 w390] -> w384
                      tunnel: w381 -> [w386 w390]
                      tunnel: w380 -> [w385 _]
                      frame "Closed" {
                        n133 = invoke class="VI" method="FP.Open"(reference=w385, error in=w386, "Activate"=TRUE, "State"=T6."Standard") -> (error out=w387:errorcluster)  [unwired: 1 in, 4 out]
                      }
                      frame Default {
                      }
                    }
                  }
                  frame "Close" {
                    n134 = property class="VI"(reference=w393, error in=w395) -> (reference out=w392:refnum<vi>, error out=w394:errorcluster, "FP.State"=w391:T6)
                    n135 = case shown="Default" w391 {
                      tunnel: [w397 w400] -> w396
                      tunnel: w394 -> [w397 w399]
                      tunnel: w392 -> [_ w398]
                      frame "Invalid", "Closed" {
                      }
                      frame Default {
                        n136 = invoke class="VI" method="FP.Close"(reference=w398, error in=w399) -> (error out=w400:errorcluster)  [unwired: 1 in, 2 out]
                      }
                    }
                  }
                }
              }
              frame condition #1 {
              }
            }
            n137 = call <vilib>:"Add State(s) to Queue__jki_lib_state_machine.vi"("State(s) in (\"\")"=w374) -> ("States Out"=w373:string)  [unwired: 14 in]
          }
          frame "UI: Send to UI" {
            w403 = T25 {"Current, A"=0.0, "Magnitude"=0.0}  # Measurement.WavelengthSweeping.Measured
            # "TODO: Add XY units, or XY array indexes?"
            n138 = Unbundle By Name(w410) -> ("Self Reference"=w409:refnum<class "Measurement.PhotocurrentMapping.lvclass">, "Results.SMU Measurement"=w408:dbl, "Results.LIA Measurement"=w407:dbl)
            n139 = Bundle By Name(cluster=w403, "Current, A"=w408, "Magnitude"=w407) -> (w406:T25)
            n140 = To Variant(anything=w406) -> (Variant=w402:variant)
            n141 = call "Measurement.OnMeasured.vi"("error in (no error)"=w405, "Payload"=w402, "Measurement in"=w409) -> ("error out"=w404:errorcluster)  [unwired: 7 in, 1 out]
            n142 = call <vilib>:"Add State(s) to Queue__jki_lib_state_machine.vi"("State(s) in (\"\")"=w413) -> ("States Out"=w412:string)  [unwired: 14 in]
          }
          frame "---------- Macro ----------" {
            # "Do not put any code in this frame.\n(It is a separator no-op. You can make a copy of this frame to create a new Macro frame)"
            n143 = call <vilib>:"Add State(s) to Queue__jki_lib_state_machine.vi"("State(s) in (\"\")"=w418) -> ("States Out"=w417:string)  [unwired: 14 in]
          }
          frame "Macro: Initialize" {
            w421 = "UI: Initialize\n//UI: Front Panel State >> Open"  # UI: Initialize //UI: Front Panel State >> Open
            # "Initialization Macro\n(This is called once, when the VI starts)"
            n144 = call <vilib>:"Add State(s) to Queue__jki_lib_state_machine.vi"("State(s) in Front (\"\")"="Data: Initialize\nInitialize Core Data\nEvents: Register\nData: Initialize Grid", "State(s) in (\"\")"="Process: Sync", "State(s) at Back (\"\")"=w421) -> ("States Out"=w420:string)  [unwired: 12 in]
            n145 = call <vilib>:"Add State(s) to Queue__jki_lib_state_machine.vi"("State(s) in Front (\"\")"=w420, "State(s) in (\"\")"=w427) -> ("States Out"=w426:string)  [unwired: 13 in]
          }
          frame "Macro: Exit" {
            # "Exit Macro\n(This is called once, when the VI exits)"
            n146 = Unbundle By Name(w432) -> ("Core.Close Panel on Exit?"=w438:bool)
            n147 = Select(t="UI: Front Panel State >> Close", s=w438, f="") -> (s? t:f=w435:string)
            n148 = call <vilib>:"Add State(s) to Queue__jki_lib_state_machine.vi"("State(s) in Front (\"\")"="Data: Cleanup\nEvents: Unregister", "State(s) in (\"\")"="Process: Sync", "State(s) at Back (\"\")"="Exit") -> ("States Out"=w429:string)  [unwired: 12 in]
            n149 = call <vilib>:"Add State(s) to Queue__jki_lib_state_machine.vi"("State(s) in (\"\")"=w435, "State(s) at Back (\"\")"=w429) -> ("States Out"=w434:string)  [unwired: 13 in]
            n150 = call <vilib>:"Add State(s) to Queue__jki_lib_state_machine.vi"("State(s) in Front (\"\")"=w434, "State(s) in (\"\")"=w441) -> ("States Out"=w440:string)  [unwired: 13 in]
          }
          frame "Macro: Measurement Start" {
            n151 = call <vilib>:"Add State(s) to Queue__jki_lib_state_machine.vi"("State(s) in Front (\"\")"="Measurement: Move\nMeasurement: Measure >> All\nUI: Send to UI\nMeasurement: Next Step", "State(s) in (\"\")"=w447) -> ("States Out"=w446:string)  [unwired: 13 in]
          }
          frame "Macro: Measurement Stop" {
            n152 = Unbundle By Name(w452) -> ("Self Reference"=w451:refnum<class "Measurement.PhotocurrentMapping.lvclass">)
            n153 = call "Measurement.OnFinished.vi"("error in (no error)"=w450, "Finished"=T7 TRUE, "Measurement in"=w451) -> ("error out"=w449:errorcluster)  [unwired: 7 in, 1 out]
            n154 = Bundle By Name(cluster=w452, "P-Map State"=Measurement.PhotocurrentMapping.State--Enum."Stoppped" ("W-Sweep State")) -> (w453:T23)
            n155 = call <vilib>:"Add State(s) to Queue__jki_lib_state_machine.vi"("State(s) in Front (\"\")"="Measurement: SMU >> Set Output Disable", "State(s) in (\"\")"="Measurement: OPA >> Set Shutter state Close") -> ("States Out"=w455:string)  [unwired: 13 in]
            n156 = call <vilib>:"Add State(s) to Queue__jki_lib_state_machine.vi"("State(s) in Front (\"\")"=w455, "State(s) in (\"\")"=w460) -> ("States Out"=w459:string)  [unwired: 13 in]
          }
          frame "---------- Process ----------" {
            # "Template Separator\n(You can make a copy of, or modify, this frame)"
            n157 = call <vilib>:"Add State(s) to Queue__jki_lib_state_machine.vi"("State(s) in (\"\")"=w465) -> ("States Out"=w464:string)  [unwired: 14 in]
          }
          frame "Process: Sync" {
            n158 = Unbundle By Name(w473) -> ("Self Reference"=w469:refnum<class "Measurement.PhotocurrentMapping.lvclass">)
            n159 = call <vilib>:"WaitOnProcessSync.vi"("error in (no error)"=w468, "SMO"=w469) -> ("error out"=w467:errorcluster, "Don't run?"=w472:bool)  [unwired: 7 in, 1 out]
            n160 = Select(t="Data: Cleanup\nEvents: Unregister\nExit", s=w472, f="") -> (s? t:f=w466:string)
            n161 = call <vilib>:"Add State(s) to Queue__jki_lib_state_machine.vi"("State(s) in Front (\"\")"=w466, "State(s) in (\"\")"=w476) -> ("States Out"=w475:string)  [unwired: 13 in]
          }
          frame "---------- Events ----------" {
            # "Template Separator\n(You can make a copy of, or modify, this frame)"
            n162 = call <vilib>:"Add State(s) to Queue__jki_lib_state_machine.vi"("State(s) in (\"\")"=w481) -> ("States Out"=w480:string)  [unwired: 14 in]
          }
          frame "Events: Register" {
            # "Static Dependencies\nPublic Events"
            # "Measurement base\nProtected events"
            # "Base Class Protected Events"
            n163 = Unbundle By Name(w485) -> ("Self Reference"=w495:refnum<class "Measurement.PhotocurrentMapping.lvclass">)
            n164 = Unbundle By Name(w485) -> ("Dependencies.XYStage"=w484:refnum<class "XYStage.lvclass">)
            n165 = Unbundle By Name(w485) -> ("Dependencies.SMU"=w493:refnum<class "SMU.lvclass">)
            n166 = Unbundle By Name(w485) -> ("Dependencies.LIA"=w492:refnum<class "LIA.lvclass">)
            n167 = call "Measurement.GetProtectedEventsRegistration.vi"("Measurement in"=w495) -> ("error out"=w489:errorcluster, "Measurement Protected Events"=w494:refnum<event-registration>)  [unwired: 8 in, 1 out]
            n168 = call <vilib>:"GetProtectedEvents.vi"("SMO"=w495) -> ("error out"=w499:errorcluster, "SMO Protected Events"=w501:T26)  [unwired: 8 in, 1 out]
            n169 = call "SMU.GetPublicEventsRegistration.vi"("SMU"=w493) -> ("error out"=w488:errorcluster, "SMU Public Events"=w491:refnum<event-registration>)  [unwired: 8 in, 1 out]
            n170 = call "LIA.GetPublicEventsRegistration.vi"("LIA"=w492) -> ("error out"=w487:errorcluster, "LIA Public Events"=w490:refnum<event-registration>)  [unwired: 8 in, 1 out]
            n171 = call "XYStage.GetPublicEventsRegistration.vi"("XYStage"=w484) -> ("error out"=w483:errorcluster, "XYStage Public Events"=w482:refnum<event-registration>)  [unwired: 8 in, 1 out]
            n172 = register-events(w501) -> (reference out=w496:refnum<event-registration>, error out=w500:errorcluster)  [unwired: 2 in]
            n173 = Bundle("Event Registration Refnum"=w496, "Measurement Protected Events"=w494, "SMU Public Events"=w491, "LIA Public Events"=w490, "XYStage Public Events"=w482) -> (w497:T27)  [unwired: 1 in]
            n174 = Merge Errors(w500, w499, w489, w488, w487, w483, w486) -> (w498:errorcluster)
            n175 = call <vilib>:"Add State(s) to Queue__jki_lib_state_machine.vi"("State(s) in (\"\")"=w503) -> ("States Out"=w502:string)  [unwired: 14 in]
          }
          frame "Events: Unregister" {
            n176 = Unregister For Events(event registration refnum=w506, error in=w505) -> (error out=w504:errorcluster)
            n177 = call <vilib>:"Clear Errors.vi"("error in (no error)"=w504) -> ()  [unwired: 5 in, 2 out]
            n178 = call <vilib>:"Add State(s) to Queue__jki_lib_state_machine.vi"("State(s) in (\"\")"=w509) -> ("States Out"=w508:string)  [unwired: 14 in]
          }
          frame "---------- API ----------" {
            n179 = call <vilib>:"Add State(s) to Queue__jki_lib_state_machine.vi"("State(s) in (\"\")"=w514) -> ("States Out"=w513:string)  [unwired: 14 in]
          }
          frame "Action: Initialize" {
            n180 = call-dynamic "Measurement.Init.vi"("error in (no error)"=w523, "Measurement.PhotocurrentMapping in"=w524) -> ("error out"=w522:errorcluster, "Result"=w515:bool, "Measurement.PhotocurrentMapping out"=w521:refnum<class "Measurement.PhotocurrentMapping.lvclass">)  [unwired: 6 in, 1 out]
            n181 = case shown="False" w515 {
              tunnel: w522 -> [w531 w534]
              tunnel: [w530 w534] -> w520
              frame False {
                n182 = call <vilib>:"Error Cluster From Error Code.vi"("error in (no error)"=w531, "error message (\"\")"="Measurement Initialization failure" ("source"), "error code (0)"=-8000 ("code")) -> ("error out"=w530:errorcluster)  [unwired: 6 in]
              }
              frame True {
              }
            }
            n183 = call "Measurement.OnInitialized.vi"("error in (no error)"=w520, "Initialized"=w515, "Measurement in"=w521) -> ("error out"=w516:errorcluster)  [unwired: 7 in, 1 out]
            n184 = case shown="True" w515 {
              tunnel: [Measurement.State--Enum."Uninitialized" ("State") Measurement.State--Enum."Initialized" ("State")] -> w517
              frame False {
              }
              frame True {
              }
            }
            n185 = Bundle By Name(cluster=w519, "Meas State"=w517, "Initialized"=w515) -> (w518:T23)
            n186 = call <vilib>:"Add State(s) to Queue__jki_lib_state_machine.vi"("State(s) in (\"\")"=w527) -> ("States Out"=w526:string)  [unwired: 14 in]
          }
          frame "Action: Uninitialize" {
            n187 = Unbundle By Name(w536) -> ("Initialized"=w535:bool)
            n188 = case shown="True" w535 {
              tunnel: w542 -> [_ w552]
              tunnel: w541 -> [w546 w551]
              tunnel: [w546 w548] -> w540
              frame False {
              }
              frame True {
                n189 = call-dynamic "Measurement.Uninit.vi"("error in (no error)"=w551, "Measurement.PhotocurrentMapping in"=w552) -> ("error out"=w549:errorcluster, "Measurement.PhotocurrentMapping out"=w550:refnum<class "Measurement.PhotocurrentMapping.lvclass">)  [unwired: 8 in]
                n190 = call "Measurement.OnUninitialized.vi"("error in (no error)"=w549, "Uninitialized (True)"=T8 TRUE ("Uninitialized"), "Measurement in"=w550) -> ("error out"=w548:errorcluster)  [unwired: 7 in, 1 out]
              }
            }
            n191 = Bundle By Name(cluster=w536, "Initialized"=FALSE, "Meas State"=Measurement.State--Enum."Uninitialized" ("State")) -> (w539:T23)
            n192 = call <vilib>:"Add State(s) to Queue__jki_lib_state_machine.vi"("State(s) in (\"\")"=w545) -> ("States Out"=w544:string)  [unwired: 14 in]
          }
          frame "Action: Escape" {
            w553 = T28 TRUE  # Escaped
            n193 = call "Measurement.OnEscaped.vi"("error in (no error)"=w555, "Escaped"=w553, "Measurement in"=w556) -> ("error out"=w554:errorcluster)  [unwired: 7 in, 1 out]
            n194 = call <vilib>:"Add State(s) to Queue__jki_lib_state_machine.vi"("State(s) in (\"\")"=w560) -> ("States Out"=w559:string)  [unwired: 14 in]
          }
        }
      }
    }
    frame Error {
    }
  }
  n195 = call-parent "Process.vi"("error in"=w8, "SMO"=w7) -> ("error out"=w5:errorcluster, "SMO out"=→"Measurement.PhotocurrentMapping out":refnum<class "Measurement.PhotocurrentMapping.lvclass">)  [unwired: 8 in]
  n196 = Merge Errors(w5, w4) -> (→"error out":errorcluster)
